vi "Popualte Names Release.vi"(8 "error in (no error)":errorcluster, 11 "ClusterConstant in":refnum<vi>) -> (0 "error out":errorcluster)   [LabVIEW 2014, in "Initialization and IO Node Scripting.lvlib"]
uses:
  Initialization and IO Node Scripting.lvlib
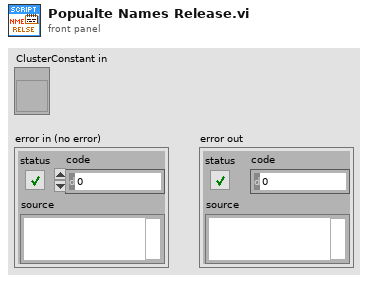
[diagram p1: front panel]
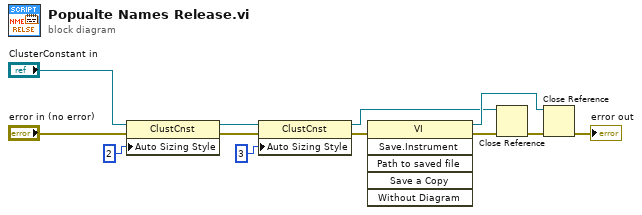
[diagram p0: block diagram]
diagram:
  n1 = property class="ClustCnst"(reference="ClusterConstant in", error in="error in (no error)", "Auto Sizing Style"=u32 2 ("Auto Sizing")) -> (reference out=w6:refnum<vi>, error out=w5:errorcluster)
  n2 = property class="ClustCnst"(reference=w6, error in=w5, "Auto Sizing Style"=u32 3 ("Auto Sizing")) -> (reference out=w2:refnum<vi>, error out=w3:errorcluster)
  n3 = invoke class="VI" method="Save.Instrument"(error in=w3) -> (reference out=w9:refnum<vi>, error out=w1:errorcluster)  [unwired: 5 in, 4 out]
  n4 = Close Reference(reference=w2, error in (no error)=w1) -> (error out=w8:errorcluster)
  n5 = Close Reference(reference=w9, error in (no error)=w8) -> (error out=→"error out":errorcluster)
